vi "iTC_Readout_bak.vi"() -> ()   [LabVIEW 2009]
panel:
  in  "stop 2":bool
  out "Heartbeat":bool
  out "Cernox Temp":string
  out "Cernox Temp":dbl(graph)
  out "Cernox Temp":dbl(slide) scale=0.0..320.0
  out "Cernox Resistance":dbl(graph)
  out "Cernox Resistance":dbl(knob) scale=0.0..300.0
  out "Cernox Resistance":string
  in  "stop":bool
  out "Measurement":bool caption="Taken"
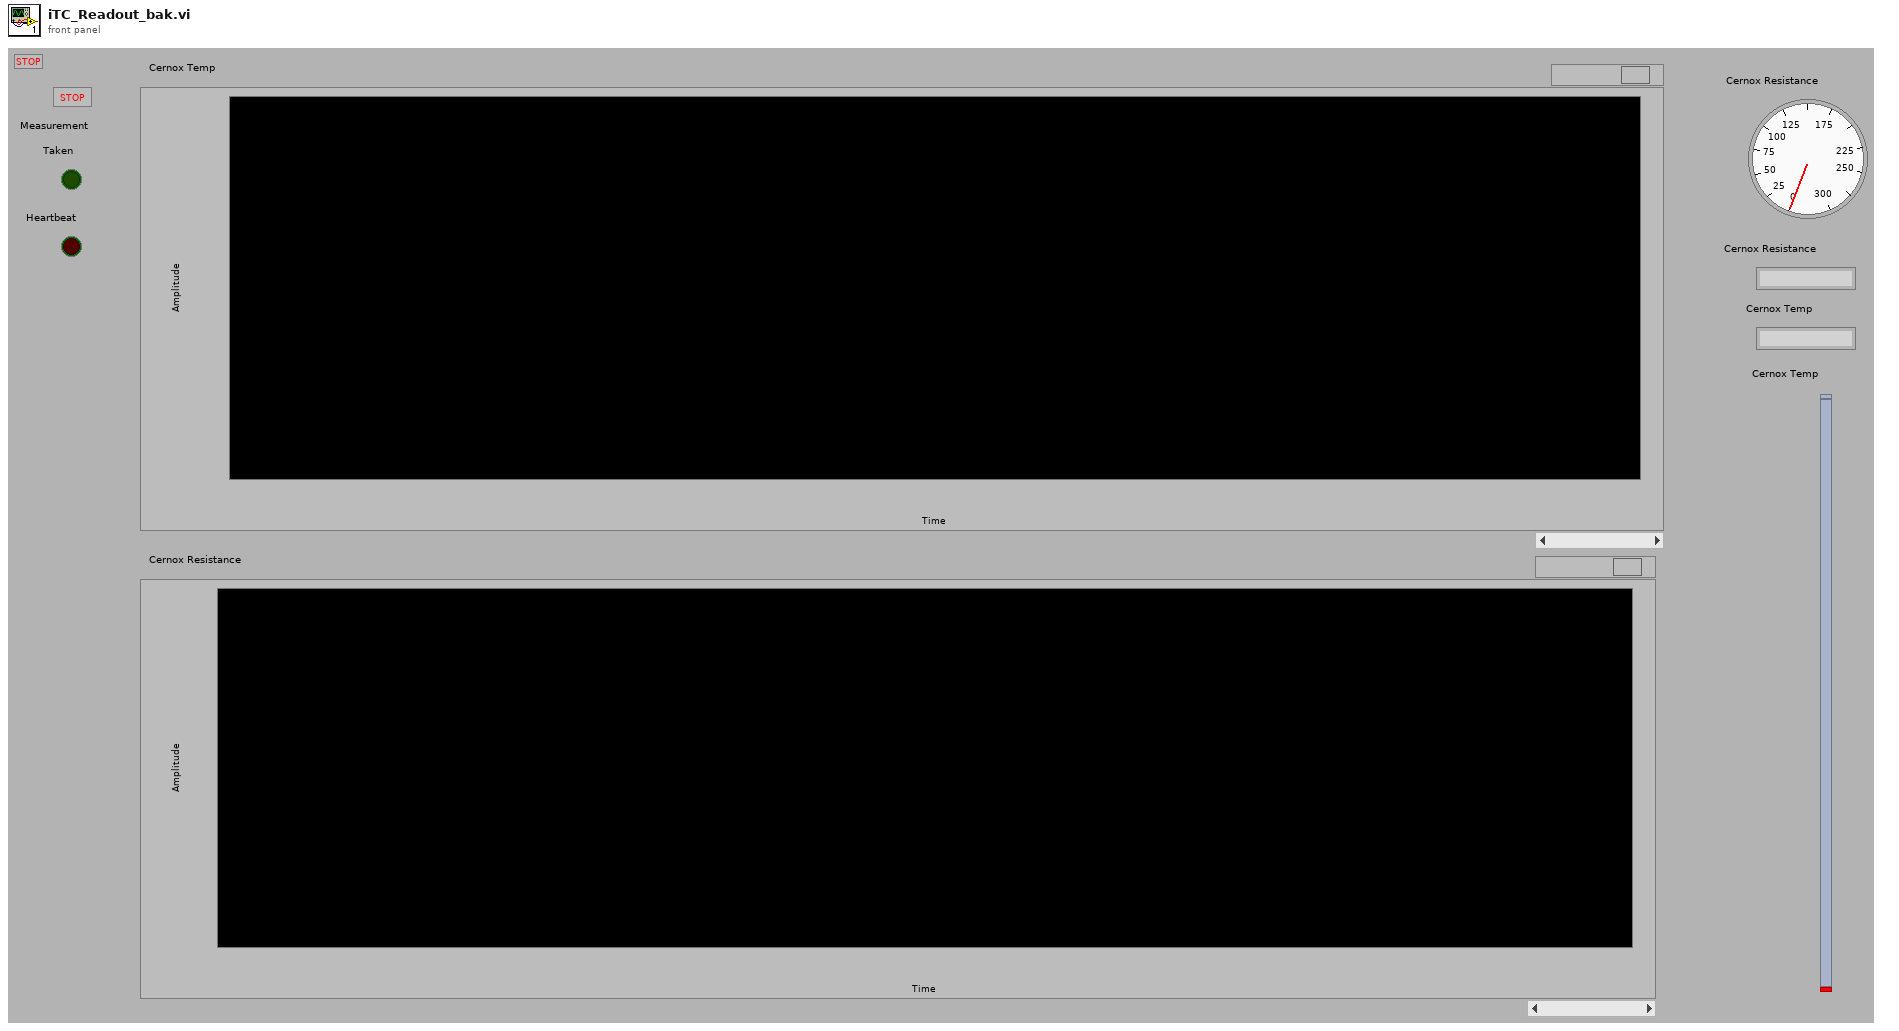
[diagram p1: front panel]
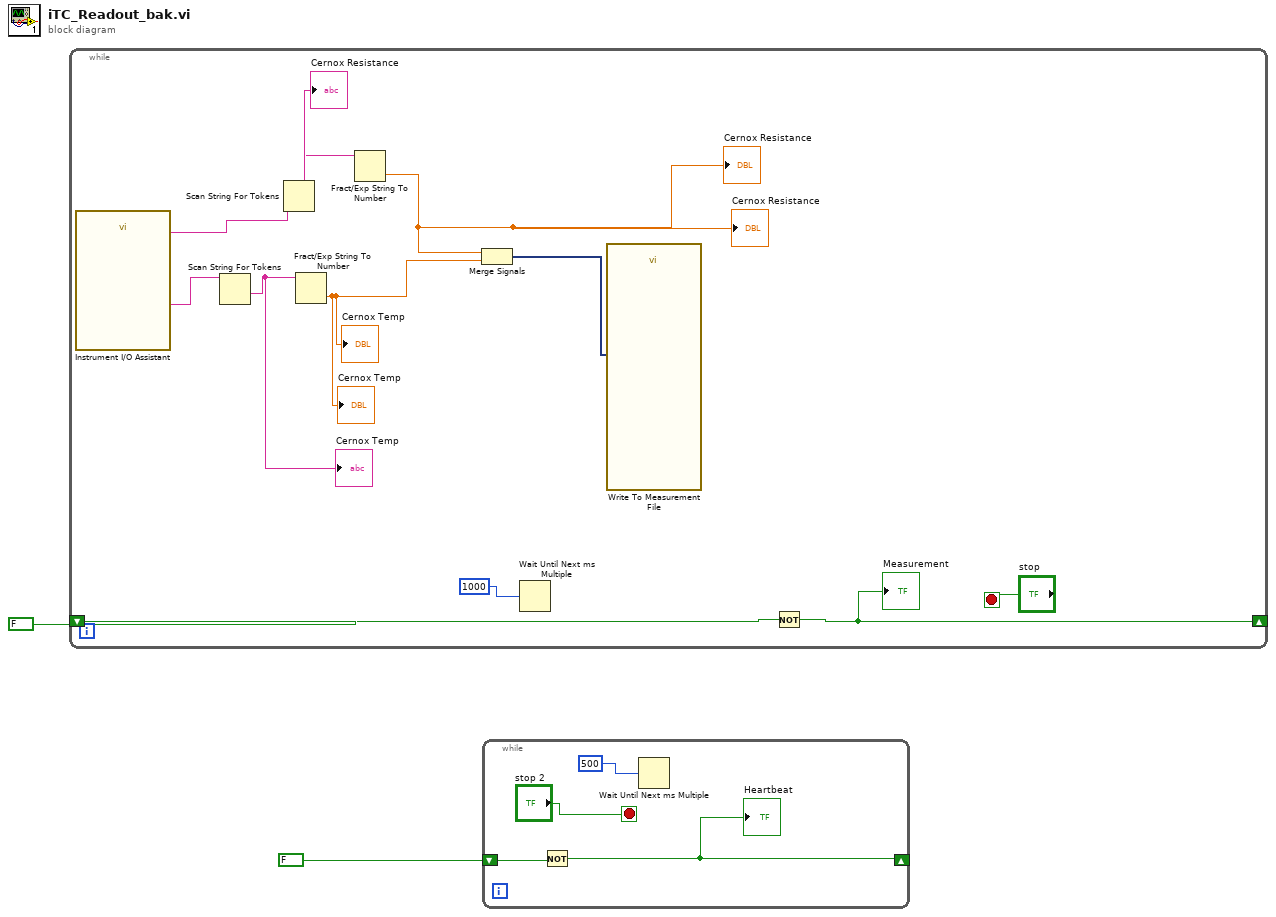
[diagram p0: block diagram]
diagram:
  n1 = while {
    shift-right: [w11] -> _
    shift-left: FALSE -> [w12]
    stop <- "stop" stop-if-true
    n2 = call "Instrument I/O Assistant"() -> ("Cernox Temp"=w7:string, "Cernox Resistance"=w9:string)  [unwired: 25 in, 1 out]
    n3 = Scan String For Tokens(9:w7) -> (1:w3:string)  [unwired: 5 in, 3 out]
    "Cernox Temp" <- w3
    n4 = Scan String For Tokens(9:w9) -> (1:w8:string, 3:→"Cernox Resistance":string)  [unwired: 5 in, 2 out]
    n5 = Fract/Exp String To Number(string=w3) -> (number=w4:dbl)  [unwired: 3 in, 1 out]
    "Cernox Temp" <- w4
    "Cernox Temp" <- w4
    n6 = Fract/Exp String To Number(string=w8) -> (number=w5:dbl)  [unwired: 3 in, 1 out]
    "Cernox Resistance" <- w5
    "Cernox Resistance" <- w5
    n7 = Merge Signals(w5, w4) -> (w6:dynamicdata)
    n8 = Wait Until Next ms Multiple(millisecond multiple=1000) -> ()  [unwired: 1 out]
    n9 = call "Write To Measurement File"("Signals"=w6) -> ()  [unwired: 16 in, 3 out]
    n10 = Not(x=w12) -> (.not. x?=w11:bool)
    "Measurement" <- w11
  }
  n11 = while {
    shift-right: [w16] -> _
    shift-left: FALSE -> [w17]
    stop <- "stop 2" stop-if-true
    n12 = Not(x=w17) -> (.not. x?=w16:bool)
    "Heartbeat" <- w16
    n13 = Wait Until Next ms Multiple(millisecond multiple=500) -> ()  [unwired: 1 out]
  }
